vi "GetImpairReports.vi"(8 "error in (no error)":errorcluster, 11 "NoPmuImpair":refnum<class "NoPmuImpairPlugin.lvclass">) -> (0 "error out":errorcluster, 3 "NoPmuImpair":refnum<class "NoPmuImpairPlugin.lvclass">)   [LabVIEW 2014, in "PmuImpairPlugins.lvlib" / "NoPmuImpairPlugin.lvclass"]
uses:
  NoPmuImpairPlugin.lvclass
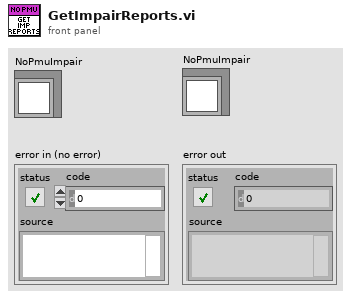
[diagram p1: front panel]
types:
  T1 = typedef "EventPlugins.lvlib/EventPluginBaseClass.lvclass/clEvtReportArray.ctl" = T2[]
  T2 = typedef "EventPlugins.lvlib/EventPluginBaseClass.lvclass/clEvtReport.ctl" = cluster{"Timestamp":dbl, "Synx":cdb[], "Freq":dbl, "ROCOF":dbl, "ID":i16}
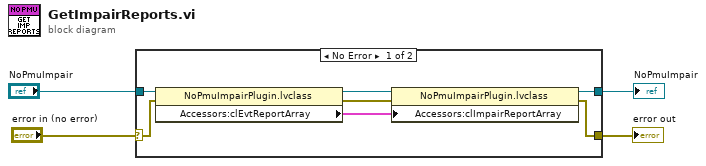
[diagram p0: block diagram]
diagram:
  n1 = case shown="No Error" "error in (no error)" {
    selector: "error in (no error)" -> [w8 w13]
    tunnel: [w6 w13] -> w3
    tunnel: [w9 w12] -> w1
    tunnel: "NoPmuImpair" -> [w11 w12]
    frame No Error {
      n2 = property class="NoPmuImpairPlugin.lvclass"(reference=w11, error in=w8) -> (reference out=w10:refnum<class "NoPmuImpairPlugin.lvclass">, error out=w5:errorcluster, "Accessors:clEvtReportArray"=w7:T1)
      n3 = property class="NoPmuImpairPlugin.lvclass"(reference=w10, error in=w5, "Accessors:clImpairReportArray"=w7) -> (reference out=w9:refnum<class "NoPmuImpairPlugin.lvclass">, error out=w6:errorcluster)
    }
    frame Error {
    }
  }
  "NoPmuImpair" <- w1
  "error out" <- w3
